vi "ELVIS III v1.1 Close AO Continuous.vi"(8 "error in (no error)":errorcluster, 10 "AO (Continuous) Channels List":T1 caption="AI (Continuous) Channels List", 11 "AO (Continuous) Ref In":T3 caption="AI (Continuous) Ref In") -> (0 "error out":errorcluster)   [LabVIEW 2021]
uses:
  <vilib>/myRIO/Common/Instrument Driver Framework/Utilities/typedefs/myRIO v1.0 Reference.ctl
  <vilib>/myRIO/Common/Instrument Driver Framework/Utilities/typedefs/Generic FPGA Reference.ctl
  <vilib>/myRIO/Common/Instrument Driver Framework/ELVIS III v1.0/AO Continuous/typedefs/AO Continuous Channels List.ctl
  <vilib>/myRIO/Common/Instrument Driver Framework/ELVIS III v1.0/AO Continuous/typedefs/ELVIS III v1.0 AO Continuous Channels Enum.ctl
  <vilib>/myRIO/Common/Instrument Driver Framework/ELVIS III v1.0/AO Continuous/vis/ELVIS III v1.0 Build MUX Configuration AO Continuous.vi
  <vilib>/myRIO/Common/Instrument Driver Framework/ELVIS III v1.0/Resource Manager/vis/ELVIS III v1.0 Unreserve Channel List.vi
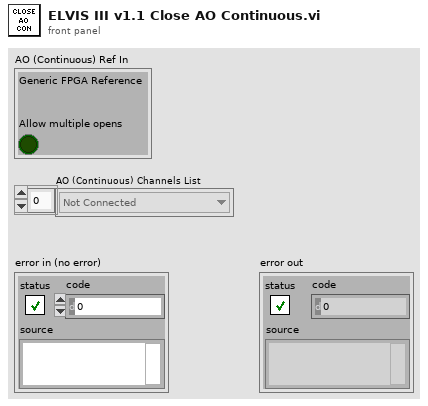
[diagram p1: front panel]
types:
  T1 = typedef "AO Continuous Channels List.ctl" = T2[]
  T2 = typedef "ELVIS III v1.0 AO Continuous Channels Enum.ctl" = enum16{"Not Connected", "A/AO0 (Continuous)", "A/AO1 (Continuous)", "B/AO0 (Continuous)", "B/AO1 (Continuous)"}
  T3 = typedef "myRIO v1.0 Reference.ctl" = cluster{"Generic FPGA Reference":T4, "Allow multiple opens":bool}
  T4 = typedef "Generic FPGA Reference.ctl" = refnum<k20>
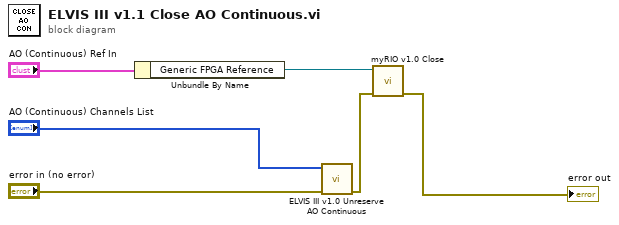
[diagram p0: block diagram]
diagram:
  n1 = Unbundle By Name("AO (Continuous) Ref In") -> ("Generic FPGA Reference"=w2:T4)
  n2 = call <vilib>:"ELVIS III v1.0 Unreserve AO Continuous.vi"("error in (no error)"="error in (no error)", "AO (Continuous) Channels List"="AO (Continuous) Channels List") -> ("error out"=w5:errorcluster)  [unwired: 9 in]
  n3 = call <vilib>:"myRIO v1.0 Close.vi"("error in (no error)"=w5, "myRIO FPGA Ref In"=w2) -> ("error out"=→"error out":errorcluster)  [unwired: 9 in]
